vi "03.3 Event-driven Message Implementation.vi"() -> ()   [LabVIEW 2019]
panel:
  in  "Generate Signal":bool
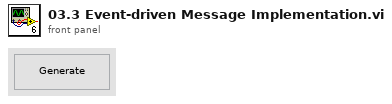
[diagram p1: front panel]
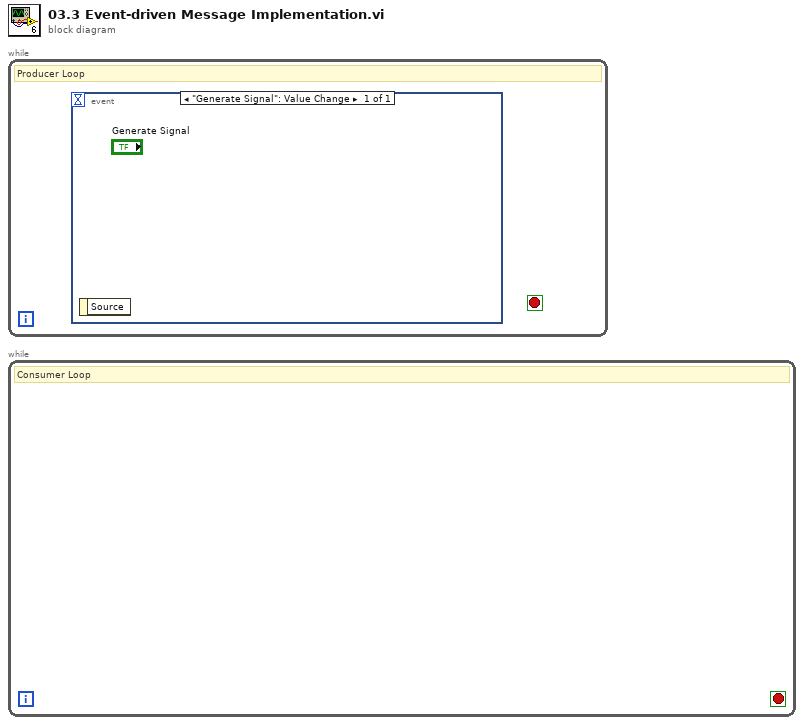
[diagram p0: block diagram]
diagram:
  n1 = while {
    stop <- _ stop-if-true
    # "Producer Loop"
    n2 = event shown="[0] \"Generate Signal\": Value Change" {
      selector: _ -> [_]
      dyn-events: _ -> [_]
      timeout: _ -> [_]
      event "Generate Signal": Value Change {
        n3 = event-data() -> ()  [unwired: 1 in, 1 out]
      }
    }
  }
  n4 = while {
    stop <- _ stop-if-true
    # "Consumer Loop"
  }
